vi "Coerce Port Power.vi"(0 "ACM4509 in":refnum<class "Cal Standard.lvclass">, 5 "Port Power":dbl, 11 "error in (no error)":errorcluster) -> (4 "ACM4509 out":refnum<class "Cal Standard.lvclass">, 6 "Coerced Port Power":dbl, 15 "error out":errorcluster)   [LabVIEW 2023, in "ACM 4509 Cal Standard.lvlib" / "Cal Standard.lvclass"]
uses:
  Cal Standard.lvclass
  C:/srd-semi-rfcal-software/AuxTools/STSRFFixtureCharactUtility/Source/Code Modules/Fixture/Instruments/Cal Standard/Cal Standard Base/Cal Standard Base.lvclass
  Properties/Read Product Name.vi
  Instruments/Cal Standard/Cal Standard Base/Cal Standard Base.lvclass
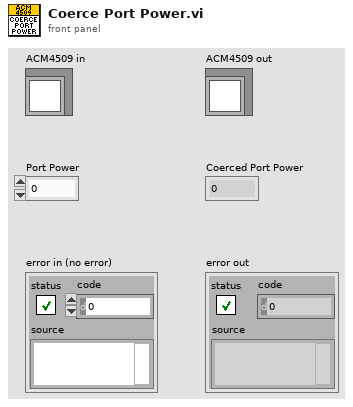
[diagram p1: front panel]
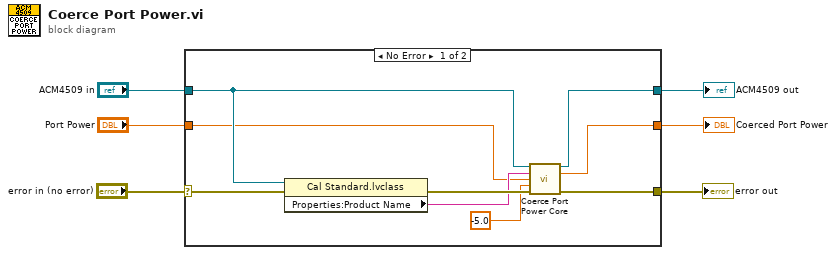
[diagram p0: block diagram]
diagram:
  n1 = case shown="No Error" "error in (no error)" {
    selector: "error in (no error)" -> [w12 w18]
    tunnel: [w15 w18] -> w1
    tunnel: [w14 w17] -> w5
    tunnel: "ACM4509 in" -> [w10 w17]
    tunnel: [w13 w16] -> w3
    tunnel: "Port Power" -> [w7 w16]
    frame No Error {
      n2 = property class="Cal Standard.lvclass"(reference=w10, error in=w12) -> (error out=w11:errorcluster, "Properties:Product Name"=w9:string)  [unwired: 1 out]
      n3 = call "Coerce Port Power Core.vi"("Cal Standard Base in"=w10, "Product Name"=w9, "Port Power"=w7, "Max Allowed Power"=-5.0 ("upper limit"), "error in (no error)"=w11) -> ("Cal Standard Base out"=w14:refnum<class "Cal Standard.lvclass">, "Coerced Port Power"=w13:dbl, "error out"=w15:errorcluster)  [unwired: 8 in]
    }
    frame Error {
    }
  }
  "error out" <- w1
  "ACM4509 out" <- w5
  "Coerced Port Power" <- w3
